vi "Interpret_Read Exception Status.vi"(8 "error in (no error)":errorcluster, 11 "MB_PDU_resp in":T1={"Function Code"=1, "Data"=[], "RTU_DataBytes"=0}) -> (0 "error out":errorcluster, 2 "Exception Status":u8)   [LabVIEW 2012, in "MB Master.lvlib"]
doc: "Extracts the data of a PDU request/response pair based on the function code of the response.\n\nReturns an array of booleans for coils and discrete inputs.\nReturns an array of unsigned 16-bit integers for input and holding registers."
uses:
  MB Master.lvlib
  MB_PDU_Cluster.ctl
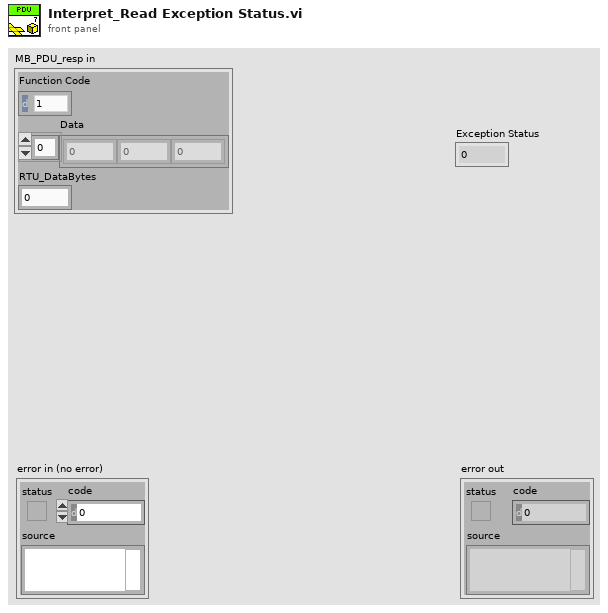
[diagram p1: front panel]
types:
  T1 = typedef "MB Master.lvlib/MB_PDU_Cluster.ctl" = cluster{"Function Code":u8, "Data":u8[], "RTU_DataBytes":i32}
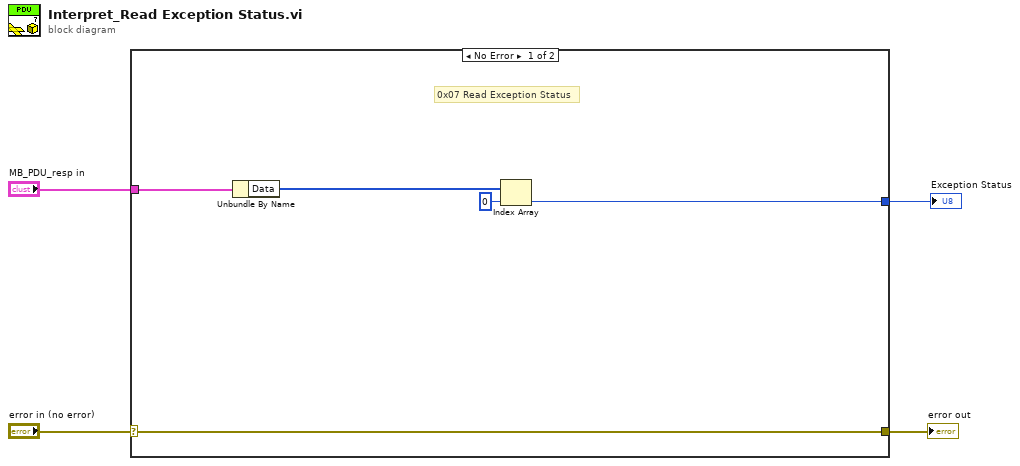
[diagram p0: block diagram]
diagram:
  n1 = case shown="No Error" "error in (no error)" {
    selector: "error in (no error)" -> [w9 w10]
    tunnel: [w9 w10] -> w3
    tunnel: "MB_PDU_resp in" -> [w8 _]
    tunnel: [w5 _] -> w1
    frame No Error {
      # "0x07 Read Exception Status"
      n2 = Unbundle By Name(w8) -> ("Data"=w7:u8[])
      n3 = Index Array(array=w7, index=0) -> (element=w5:u8)
    }
    frame Error {
    }
  }
  "error out" <- w3
  "Exception Status" <- w1
